vi "SetFilter.vi"(7 "Filter":T1=enum."NoFilter", 8 "a":dbl[](array[numeric]), 9 "b":dbl[](array[numeric]), 10 "Gain":dbl, 11 "SamplingFrequency":dbl) -> (3 "SetFilterMessage":string)   [LabVIEW 2019]
uses:
  FilterTypeDef.ctl
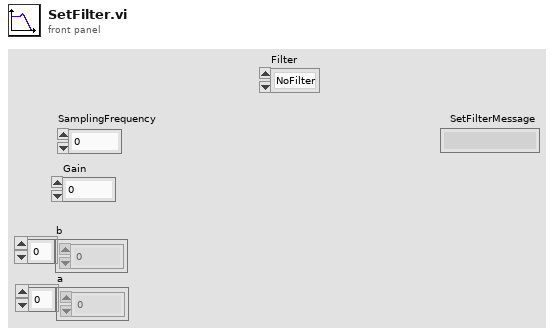
[diagram p1: front panel]
types:
  T1 = typedef "FilterTypeDef.ctl" = enum16{"IIR_X", "IIR_Y", "NoFilter", "Bessel6thOrder300"}
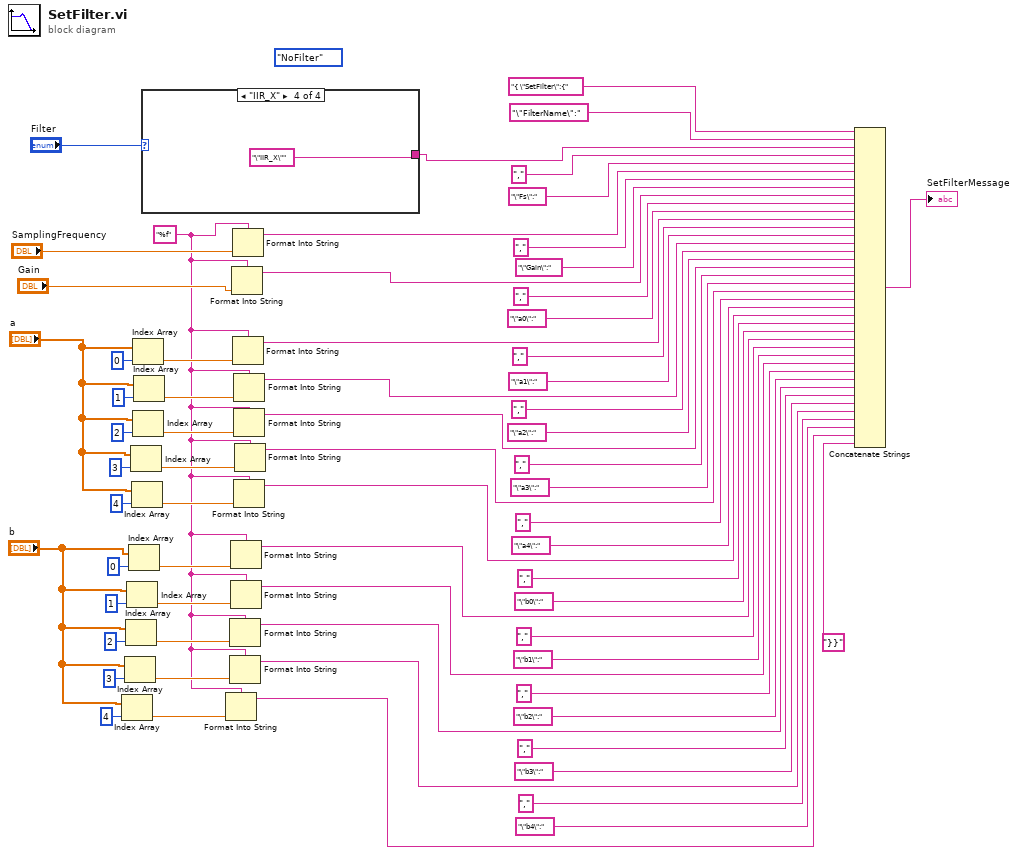
[diagram p0: block diagram]
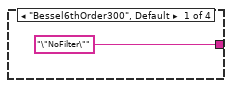
[diagram p2: hidden frame]
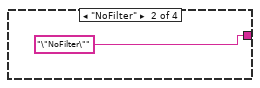
[diagram p3: hidden frame]
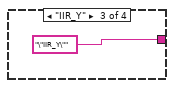
[diagram p4: hidden frame]
diagram:
  w24 = "%f" ("initial string")
  (unwired) FilterTypeDef."NoFilter"
  n1 = Index Array(array="b", index=4) -> (element=w25:dbl)
  n2 = Index Array(array="b", index=3) -> (element=w26:dbl)
  n3 = Index Array(array="b", index=2) -> (element=w27:dbl)
  n4 = Index Array(array="b", index=1) -> (element=w28:dbl)
  n5 = Index Array(array="b", index=0) -> (element=w29:dbl)
  n6 = Index Array(array="a", index=3) -> (element=w31:dbl)
  n7 = Index Array(array="a", index=4) -> (element=w30:dbl)
  n8 = Index Array(array="a", index=0) -> (element=w46:dbl)
  n9 = Index Array(array="a", index=2) -> (element=w32:dbl)
  n10 = Index Array(array="a", index=1) -> (element=w33:dbl)
  n11 = case shown="\"IIR_X\"" "Filter" {
    tunnel: ["\"NoFilter\"" "\"NoFilter\"" "\"IIR_Y\"" "\"IIR_X\""] -> w48
    frame "Bessel6thOrder300", Default {
    }
    frame "NoFilter" {
    }
    frame "IIR_Y" {
    }
    frame "IIR_X" {
    }
  }
  n12 = Format Into String(format string=w24, w25) -> (resulting string=w17:string)  [unwired: 2 in, 1 out]
  n13 = Format Into String(format string=w24, w27) -> (resulting string=w11:string)  [unwired: 2 in, 1 out]
  n14 = Format Into String(format string=w24, w26) -> (resulting string=w14:string)  [unwired: 2 in, 1 out]
  n15 = Format Into String(format string=w24, w29) -> (resulting string=w5:string)  [unwired: 2 in, 1 out]
  n16 = Format Into String(format string=w24, w28) -> (resulting string=w8:string)  [unwired: 2 in, 1 out]
  n17 = Format Into String(format string=w24, "Gain") -> (resulting string=w57:string)  [unwired: 2 in, 1 out]
  n18 = Format Into String(format string=w24, "SamplingFrequency") -> (resulting string=w60:string)  [unwired: 2 in, 1 out]
  n19 = Format Into String(format string=w24, w46) -> (resulting string=w54:string)  [unwired: 2 in, 1 out]
  n20 = Format Into String(format string=w24, w33) -> (resulting string=w51:string)  [unwired: 2 in, 1 out]
  n21 = Format Into String(format string=w24, w32) -> (resulting string=w23:string)  [unwired: 2 in, 1 out]
  n22 = Format Into String(format string=w24, w30) -> (resulting string=w2:string)  [unwired: 2 in, 1 out]
  n23 = Format Into String(format string=w24, w31) -> (resulting string=w20:string)  [unwired: 2 in, 1 out]
  n24 = Concatenate Strings("{ \"SetFilter\":{", "\"FilterName\":", w48, ",", "\"Fs\":", w60, ",", "\"Gain\":", w57, ",", "\"a0\":", w54, ",", "\"a1\":", w51, ",", "\"a2\":", w23, ",", "\"a3\":", w20, ",", "\"a4\":", w2, ",", "\"b0\":", w5, ",", "\"b1\":", w8, ",", "\"b2\":", w11, ",", "\"b3\":", w14, ",", "\"b4\":", w17, "}}" ("string")) -> (→"SetFilterMessage":string)
